vi "Search DQMH Module name from selection.vi"(11 "Search Module Name":string="\\Panther Dashboard for DQMH.lvproj\\Coins.lvlib\\Broadcast\\Error Reported") -> (3 "Module Name":string)   [LabVIEW 2020, in "Panther Dashboard.lvlib"]
uses:
  Panther Dashboard.lvlib
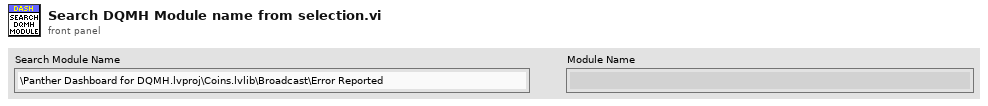
[diagram p1: front panel]
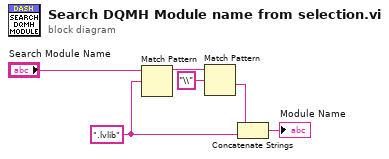
[diagram p0: block diagram]
diagram:
  w5 = ".lvlib" ("regular expression")
  n1 = Match Pattern(string="Search Module Name", regular expression=w5) -> (before substring=w3:string)  [unwired: 1 in, 3 out]
  n2 = Match Pattern(string=w3, regular expression="\\") -> (after substring=w1:string)  [unwired: 1 in, 3 out]
  n3 = Concatenate Strings(w1, w5) -> (→"Module Name":string)
